vi "Error_manager.vi"(8 "error in (no error)":errorcluster, 10 "Caller VI":refnum<vi>, 11 "Toolbox in":refnum<class "Toolbox.lvclass">) -> (0 "error out":errorcluster, 1 "source":string, 2 "code":i32, 3 "Toolbox out":refnum<class "Toolbox.lvclass">, 5 "Step":string)   [LabVIEW 2014, in "Driver_interaction.lvlib" / "Toolbox.lvclass"]
uses:
  Toolbox.lvclass
  _Driver_interaction/_Driver_interaction.lvclass/_Driver_interaction.ctl
  _Driver_interaction/_Driver_interaction.lvclass
  Deploy/Utilities/Miscelanous.lvlibp
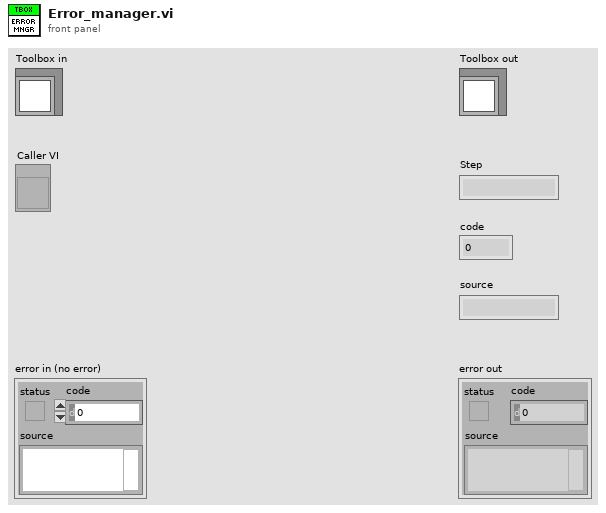
[diagram p1: front panel]
types:
  T1 = typedef "Driver_interaction.lvlib/_Driver_interaction.lvclass/Interface_type.ctl" = string
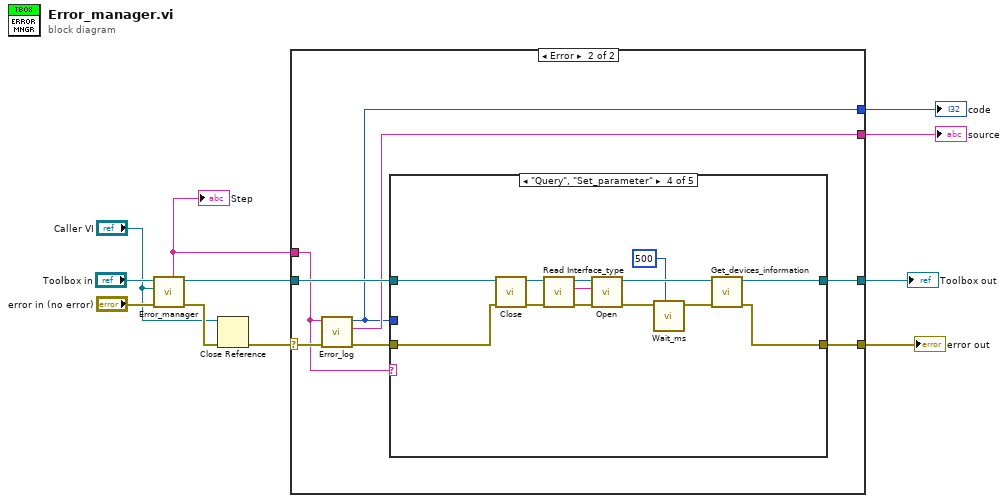
[diagram p0: block diagram]
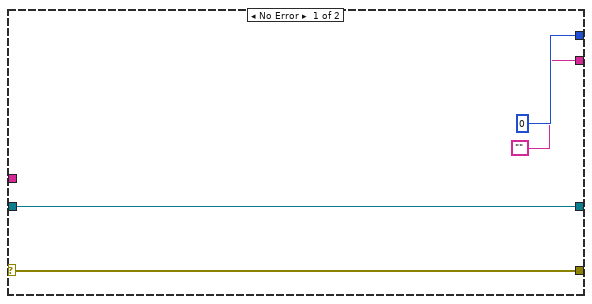
[diagram p2: hidden frame]
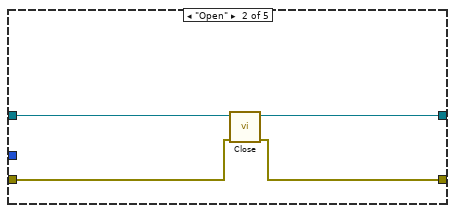
[diagram p4: hidden frame]
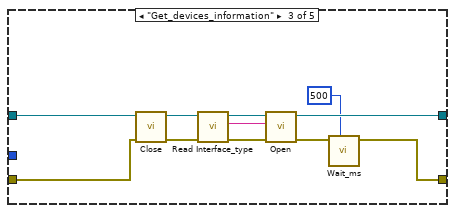
[diagram p5: hidden frame]
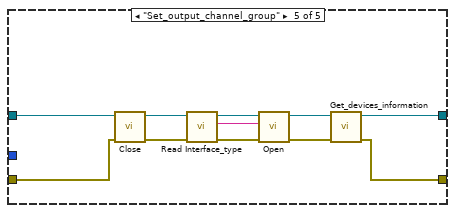
[diagram p6: hidden frame]
diagram:
  n1 = call-parent "Error_manager.vi"("error in (no error)"="error in (no error)", "Caller VI"="Caller VI", "_Driver_interaction in"="Toolbox in") -> ("error out"=w8:errorcluster, "_Driver_interaction out"=w5:refnum<class "Toolbox.lvclass">, "Step"=w2:string)  [unwired: 4 in, 2 out]
  "Step" <- w2
  n2 = Close Reference(reference="Caller VI", error in (no error)=w8) -> (error out=w9:errorcluster)
  n3 = case shown="Error" w9 {
    selector: w9 -> [w15 w23]
    tunnel: w2 -> [_ w16]
    tunnel: w5 -> [w14 w21]
    tunnel: [w14 w20] -> w6
    tunnel: [w15 w19] -> w7
    tunnel: [0 ("code") w17] -> w4
    tunnel: ["" w18] -> w3
    frame No Error {
    }
    frame Error {
      n4 = call "Error_log.vi"("error in (no error)"=w23, "Step"=w16) -> ("error out"=w22:errorcluster, "source"=w18:string, "code"=w17:i32)  [unwired: 7 in]
      n5 = case shown="\"Query\", \"Set_parameter\"" w16 {
        tunnel: w22 -> [w28 w32 w45 w51 w61]
        tunnel: w17 -> [w27 _ _ _ _]
        tunnel: w21 -> [w26 w34 w44 w58 w69]
        tunnel: [w25 w33 w43 w49 w59] -> w20
        tunnel: [w24 w31 w35 w50 w60] -> w19
        frame Default {
          # "If the issue is triggered in \"Step_name\" method"
          n6 = case shown="Default" w27 {
            tunnel: w28 -> [w29]
            tunnel: w26 -> [w30]
            tunnel: [w30] -> w25
            tunnel: [w29] -> w24
            frame Default {
              # "Create specific solutions to error code"
            }
          }
        }
        frame "Open" {
          n7 = call-dynamic "Close.vi"("error in (no error)"=w32, "Toolbox in"=w34) -> ("error out"=w31:errorcluster, "Toolbox out"=w33:refnum<class "Toolbox.lvclass">)  [unwired: 8 in]
        }
        frame "Get_devices_information" {
          n8 = call-dynamic "Close.vi"("error in (no error)"=w45, "Toolbox in"=w44) -> ("error out"=w41:errorcluster, "Toolbox out"=w42:refnum<class "Toolbox.lvclass">)  [unwired: 8 in]
          n9 = call "Read Interface_type.vi"("error in (no error)"=w41, "_Driver_interaction in"=w42) -> ("error out"=w38:errorcluster, "Interface_type"=w39:T1, "_Driver_interaction out"=w40:refnum<class "Toolbox.lvclass">)  [unwired: 7 in]
          n10 = call-dynamic "Open.vi"("error in (no error)"=w38, "Interface_type"=w39, "Toolbox in"=w40) -> ("error out"=w36:errorcluster, "Toolbox out"=w43:refnum<class "Toolbox.lvclass">)  [unwired: 7 in]
          n11 = call "Wait_ms.vi"("ms to wait"=u32 500, "error in (no error)"=w36) -> ("error out"=w35:errorcluster)  [unwired: 9 in]
        }
        frame "Query", "Set_parameter" {
          n12 = call-dynamic "Close.vi"("error in (no error)"=w51, "Toolbox in"=w58) -> ("error out"=w52:errorcluster, "Toolbox out"=w57:refnum<class "Toolbox.lvclass">)  [unwired: 8 in]
          n13 = call "Read Interface_type.vi"("error in (no error)"=w52, "_Driver_interaction in"=w57) -> ("error out"=w54:errorcluster, "Interface_type"=w53:T1, "_Driver_interaction out"=w56:refnum<class "Toolbox.lvclass">)  [unwired: 7 in]
          n14 = call-dynamic "Open.vi"("error in (no error)"=w54, "Interface_type"=w53, "Toolbox in"=w56) -> ("error out"=w48:errorcluster, "Toolbox out"=w55:refnum<class "Toolbox.lvclass">)  [unwired: 7 in]
          n15 = call "Wait_ms.vi"("ms to wait"=u32 500, "error in (no error)"=w48) -> ("error out"=w47:errorcluster)  [unwired: 9 in]
          n16 = call-dynamic "Get_devices_information.vi"("error in (no error)"=w47, "Toolbox in"=w55) -> ("error out"=w50:errorcluster, "Toolbox out"=w49:refnum<class "Toolbox.lvclass">)  [unwired: 7 in, 1 out]
        }
        frame "Set_output_channel_group" {
          n17 = call-dynamic "Close.vi"("error in (no error)"=w61, "Toolbox in"=w69) -> ("error out"=w62:errorcluster, "Toolbox out"=w68:refnum<class "Toolbox.lvclass">)  [unwired: 8 in]
          n18 = call "Read Interface_type.vi"("error in (no error)"=w62, "_Driver_interaction in"=w68) -> ("error out"=w64:errorcluster, "Interface_type"=w63:T1, "_Driver_interaction out"=w67:refnum<class "Toolbox.lvclass">)  [unwired: 7 in]
          n19 = call-dynamic "Open.vi"("error in (no error)"=w64, "Interface_type"=w63, "Toolbox in"=w67) -> ("error out"=w65:errorcluster, "Toolbox out"=w66:refnum<class "Toolbox.lvclass">)  [unwired: 7 in]
          n20 = call-dynamic "Get_devices_information.vi"("error in (no error)"=w65, "Toolbox in"=w66) -> ("error out"=w60:errorcluster, "Toolbox out"=w59:refnum<class "Toolbox.lvclass">)  [unwired: 7 in, 1 out]
        }
      }
    }
  }
  "error out" <- w7
  "Toolbox out" <- w6
  "code" <- w4
  "source" <- w3
